vi "分解数据.vi"(7 "error IO":errorcluster, 8 "滑动杆":i16(slide) scale=3.5..18.0, 9 "地图":refnum<k7>(container) caption="网页浏览器", 10 "data":string, 11 "时间":timestamp) -> (0 "uid":i16, 1 "定位":bool, 2 "纬度显示":string, 3 "经度显示":string, 4 "错误输出":errorcluster, 5 "温度":sgl, 6 "待写入的簇":T1 {"记录时间" format="%<%H:%M:%S\n%Y/%m/%d>T"})   [LabVIEW 2018]
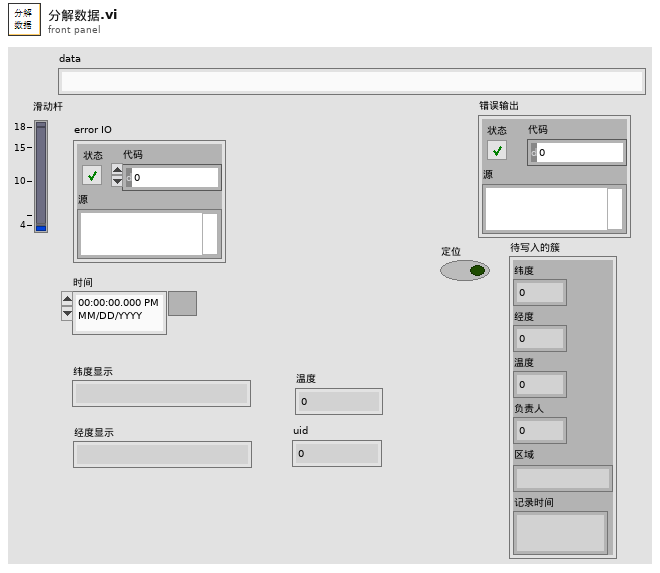
[diagram p1: front panel]
types:
  T1 = typedef "储运信息.ctl" = cluster{"纬度":sgl, "经度":sgl, "温度":sgl, "负责人":i32, "区域":string, "记录时间":timestamp}
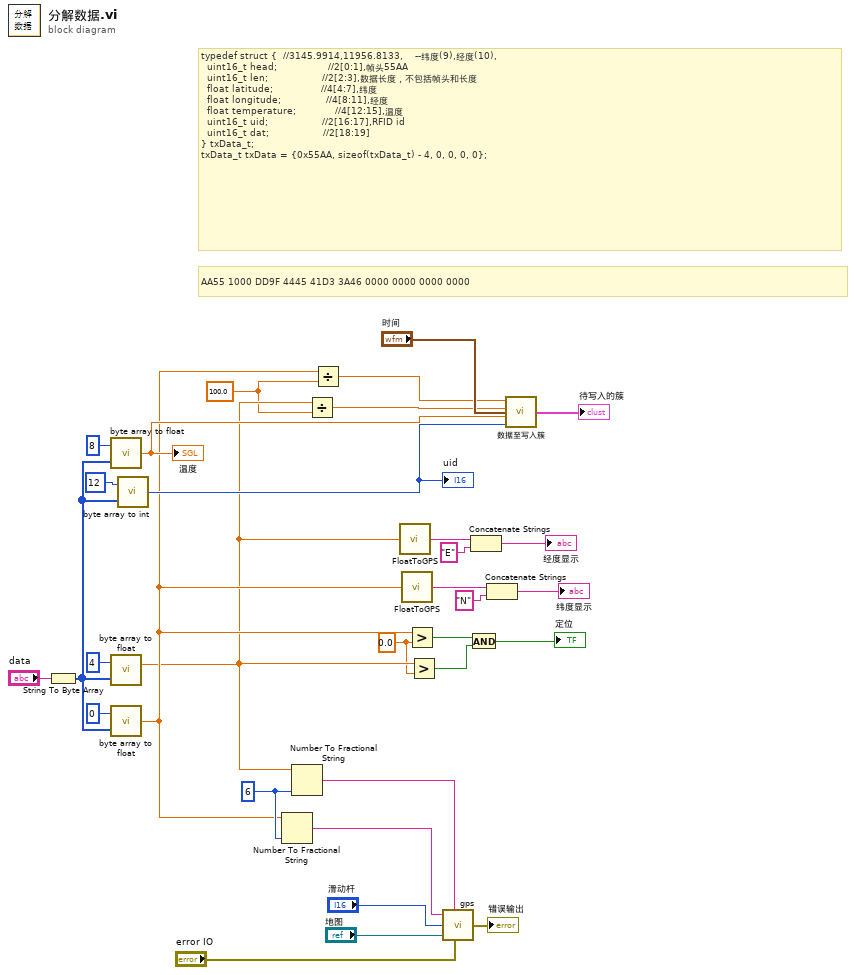
[diagram p0: block diagram]
diagram:
  w1 = sgl 0.0 ("y")
  w2 = sgl 100.0 ("y")
  w21 = i16 6 ("精度(6)")
  # "AA55 1000 DD9F 4445 41D3 3A46 0000 0000 0000 0000"
  # "typedef struct {  //3145.9914,11956.8133,    --纬度(9),经度(10),\n  uint16_t head;                 //2[0:1],帧头55AA\n  uint16_t len;                  //2[2:3],数据长度，不包括帧头和长度\n  float latitude;                //4[4:7],纬度\n  float longitude;               //4[8:11],经度\n  float temperature;             //4[12:15],温度\n  uint16_t uid;                  //2[16:17],RFID id\n  uint16_t dat;                  //2[18:19]\n} txData_t;\ntxData_t txData = {0x55AA, sizeof(txData_t) - 4, 0, 0, 0, 0};"
  n1 = String To Byte Array(string="data") -> (unsigned byte array=w26:u8[])
  n2 = call "byte array to float.vi"("unsigned byte array"=w26, "索引"=8) -> ("数值"=w10:sgl)
  "温度" <- w10
  n3 = call "byte array to float.vi"("unsigned byte array"=w26, "索引"=4) -> ("数值"=w4:sgl)
  n4 = call "byte array to float.vi"("unsigned byte array"=w26, "索引"=0) -> ("数值"=w6:sgl)
  n5 = call "byte array to int.vi"("unsigned byte array"=w26, "索引"=12) -> ("数值"=w9:i16)
  "uid" <- w9
  n6 = Number To Fractional String(number=w6, precision (6)=w21) -> (F-format string=w14:string)  [unwired: 2 in]
  n7 = Number To Fractional String(number=w4, precision (6)=w21) -> (F-format string=w13:string)  [unwired: 2 in]
  n8 = Divide(x=w4, y=w2) -> (x/y=w3:sgl)
  n9 = Divide(x=w6, y=w2) -> (x/y=w5:sgl)
  n10 = call "FloatToGPS.vi"("数字"=w4) -> ("string"=w20:string)
  n11 = call "FloatToGPS.vi"("数字"=w6) -> ("string"=w22:string)
  n12 = Greater?(x=w6, y=w1) -> (0:w30:bool)
  n13 = Greater?(x=w4, y=w1) -> (0:w31:bool)
  n14 = call "gps.vi"("纬度"=w14, "经度"=w13, "滑动杆"="滑动杆", "地图"="地图", "error IO"="error IO") -> ("错误输出"=→"错误输出":errorcluster)
  n15 = And(x=w30, y=w31) -> (x .and. y?=→"定位":bool)
  n16 = Concatenate Strings(w20, "E" ("字符串")) -> (→"经度显示":string)
  n17 = Concatenate Strings(w22, "N" ("字符串")) -> (→"纬度显示":string)
  n18 = call "数据至写入簇.vi"("纬度"=w5, "经度"=w3, "温度"=w10, "编号"=w9, "时间"="时间") -> ("数据写入"=→"待写入的簇":T1)
